vi "CheckForExtension.vi"(11 "selected path":path) -> (3 "dup file":path)   [LabVIEW 2021]
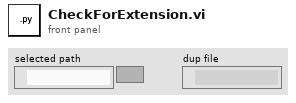
[diagram p1: front panel]
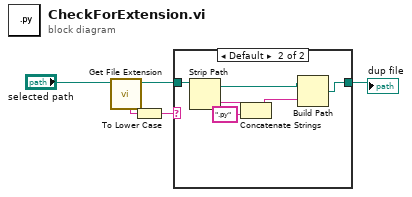
[diagram p0: block diagram]
diagram:
  n1 = call <vilib>:"Get File Extension.vi"("file"="selected path") -> ("dup file"=w3:path, "unmodified file extension"=w4:string)  [unwired: 6 in, 3 out]
  n2 = To Lower Case(string=w4) -> (all lower case string=w1:string)
  n3 = case shown="Default" w1 {
    tunnel: w3 -> [w6 w12]
    tunnel: [w6 w10] -> w2
    frame "py" {
    }
    frame Default {
      n4 = Strip Path(path=w12) -> (stripped path=w11:path, name=w9:string)
      n5 = Concatenate Strings(w9, ".py" ("string")) -> (w7:string)
      n6 = Build Path(base path=w11, name or relative path=w7) -> (appended path=w10:path)
    }
  }
  "dup file" <- w2
